vi "DeleteEntry_Http.vi"(8 "error in (no error)":errorcluster, 11 "LotData in":refnum<class "LotData.lvclass">) -> (0 "error out":errorcluster, 3 "LotData out":refnum<class "LotData.lvclass">)   [LabVIEW 2012, in "LotData.lvclass"]
uses:
  LotData.lvclass
  <vilib>/addons/database/Auxilliary.llb/DB Tools Parameter Info.ctl
  <vilib>/addons/database/Auxilliary.llb/DB Tools DataTypes.ctl
  <vilib>/addons/database/Auxilliary.llb/DB Tools Parameter Dir.ctl
  LotData.lvclass/LotData.ctl
  <vilib>/addons/database/Connection.llb/DB Tools Open Connec (Path).vi
  <vilib>/addons/database/Command.llb/Cmd Set Parameter Value (C).vi
  <vilib>/addons/database/Command.llb/Cmd Execute.vi
  <vilib>/addons/database/Recordset.llb/Rec Destroy - Command.vi
  <vilib>/addons/database/Command.llb/Cmd Delete.vi
  <vilib>/addons/database/NI_Database_API.lvlib
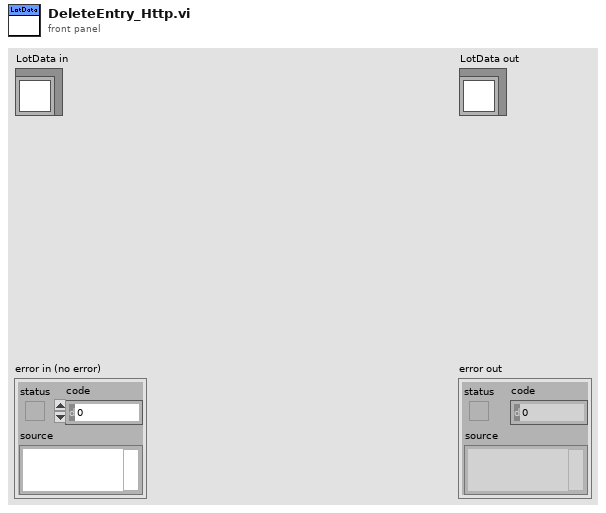
[diagram p1: front panel]
types:
  T1 = typedef "NI_Database_API.lvlib/DB Tools Parameter Info.ctl" = cluster{"parameter name":string, "type":T2, "direction":T3, "value":variant}
  T2 = typedef "NI_Database_API.lvlib/DB Tools DataTypes.ctl" = enum16{"String", "Long (I32)", "Single (SGL)", "Double (DBL)", "Date/Time", "Binary"}
  T3 = typedef "NI_Database_API.lvlib/DB Tools Parameter Dir.ctl" = enum32{"Input", "Output", "Input/Output", "Return Value"}
  T4 = typedef "NI_Database_API.lvlib/Conn ObjectReference.ctl" = refnum<k1>
  T5 = typedef "NI_Database_API.lvlib/Cmd ObjectReference.ctl" = refnum<k1>
  T6 = typedef "NI_Database_API.lvlib/Cmd-Rec Object Reference.ctl" = refnum<k1>
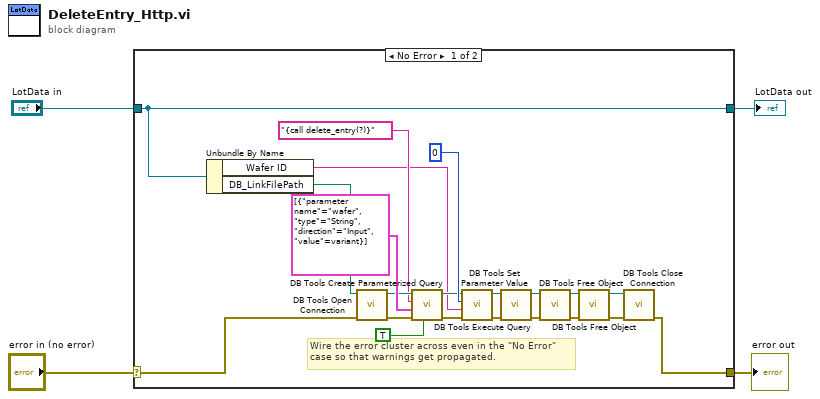
[diagram p0: block diagram]
diagram:
  n1 = case shown="No Error" "error in (no error)" {
    selector: "error in (no error)" -> [w6 w27]
    tunnel: [w7 w27] -> w3
    tunnel: [w5 w26] -> w1
    tunnel: "LotData in" -> [w5 w26]
    frame No Error {
      # "Wire the error cluster across even in the \"No Error\"\ncase so that warnings get propagated."
      n2 = Unbundle By Name(w5) -> ("Wafer ID"=w9:string, "DB_LinkFilePath"=w8:path)
      n3 = call-poly <vilib>:"DB Tools Open Connection.vi"("error in (no error)"=w6, "connection information"=w8) -> ("error out"=w22:errorcluster, "connection reference"=w23:T4)  [unwired: 6 in]
      n4 = call <vilib>:"DB Tools Create Parameterized Query.vi"("stored procedure? (F)"=TRUE, "error in (no error)"=w22, "parameters"=T1[] [{"parameter name"="wafer", "type"=enum."String", "direction"=enum."Input", "value"=variant}], "SQL query"="{call delete_entry(?)}", "connection reference"=w23) -> ("error out"=w19:errorcluster, "command reference"=w18:T5)  [unwired: 2 in, 1 out]
      n5 = call-poly <vilib>:"DB Tools Set Parameter Value.vi"("error in (no error)"=w19, "value"=w9, "parameter index"=0, "command reference"=w18) -> ("error out"=w14:errorcluster, "command reference out"=w15:T5)  [unwired: 4 in]
      n6 = call-poly <vilib>:"DB Tools Execute Query.vi"("error in (no error)"=w14, "command reference"=w15) -> ("error out"=w13:errorcluster, "command-recordset reference"=w16:T6)  [unwired: 6 in]
      n7 = call-poly <vilib>:"DB Tools Free Object.vi"("error in (no error)"=w13, "command-recordset reference"=w16) -> ("error out"=w17:errorcluster, "command reference"=w10:T5)  [unwired: 8 in]
      n8 = call-poly <vilib>:"DB Tools Free Object.vi"("error in (no error)"=w17, "command reference"=w10) -> ("error out"=w11:errorcluster, "connection reference"=w12:T4)  [unwired: 8 in]
      n9 = call <vilib>:"DB Tools Close Connection.vi"("error in (no error)"=w11, "connection reference"=w12) -> ("error out"=w7:errorcluster)  [unwired: 5 in]
    }
    frame Error {
    }
  }
  "error out" <- w3
  "LotData out" <- w1
